vi "pf_Config_and_Grab.vi"() -> ()   [LabVIEW 2012]
uses:
  <userlib>/Photonfocus Toolkit/_Public/SubVIs/pf_Set_Camera_Property_Float.vi
  <userlib>/Photonfocus Toolkit/_Public/SubVIs/pf_Set_Camera_Property_Mode.vi
  <userlib>/Photonfocus Toolkit/_Public/SubVIs/pf_Set_Camera_Property_Int.vi
  <userlib>/Photonfocus Toolkit/Photonfocus_Toolkit.lvlib
panel:
  in  "stop":bool
  in  "Tab Control":enum32{"Instructions", "image"}(tab)
  in  "Interface Name":string="img0::0||port0"
  out "Image":T1(plugin-control)
  # "1 - Open MAX and specify the correct .icd file."
  # "2 - Get the interface name from MAX (e.g: \"imag0\") and write it in the following text field. \n\n3 - Add \"::\" and the Port number showed in MAX.\n\n4 - Add \"||\" and the port name showed in PFRemote."
  # "::"
  # "||port0"
  # "Example:   img0::0||port0"
  # "5 - Close MAX before start grabbing"
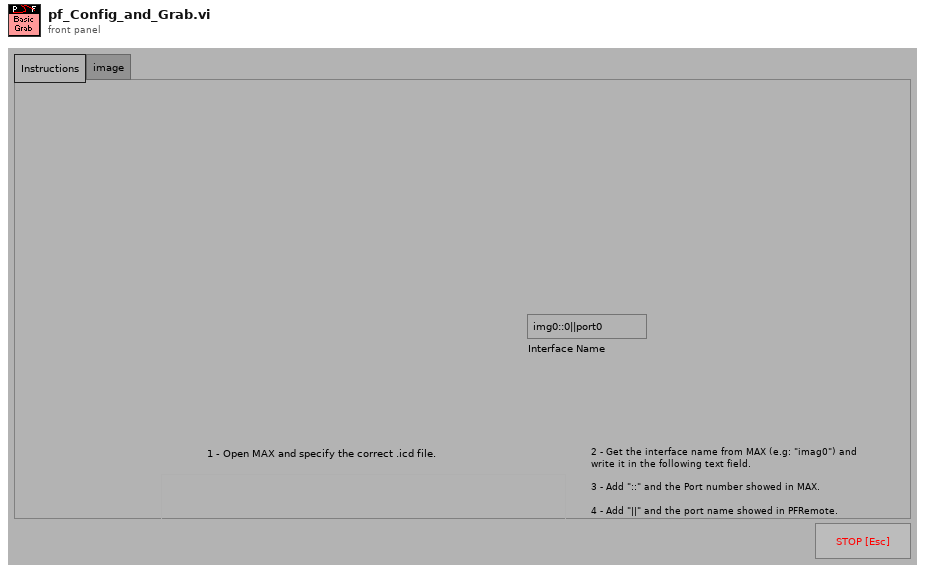
[diagram p1: front panel]
types:
  T1 = typedef "IMAQ Image.ctl" = refnum<image>
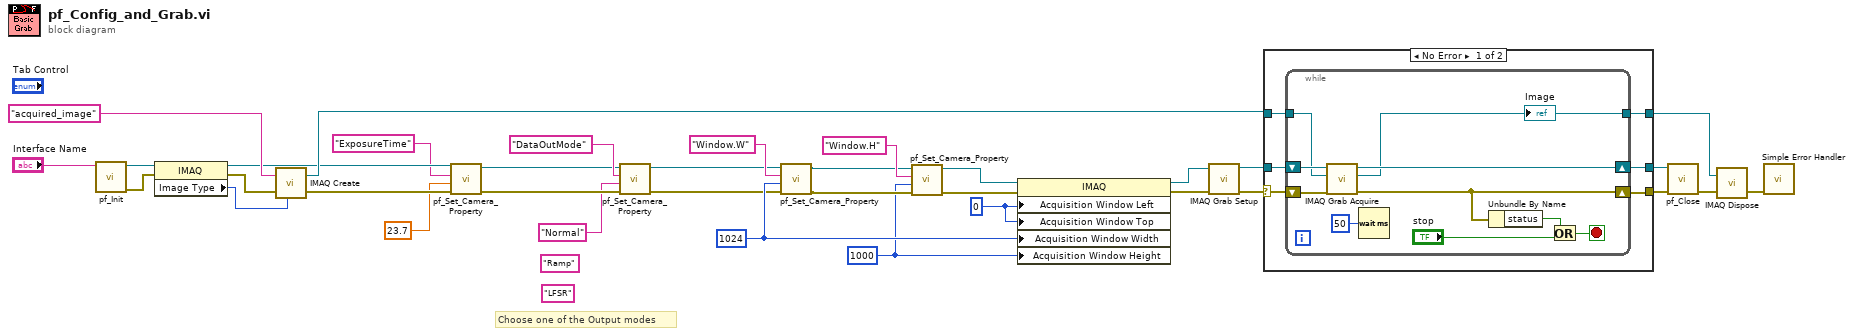
[diagram p0: block diagram]
diagram:
  w1 = u32 1000 ("milliseconds to wait")
  w15 = u32 0 ("milliseconds to wait")
  (unwired) "Ramp" ("Property Value")
  (unwired) "LFSR" ("Property Value")
  w7 = u32 1024 ("milliseconds to wait")
  # "Choose one of the Output modes"
  n1 = call <userlib>:"pf_Init.vi"("Interface Name"="Interface Name") -> ("error out"=w28:errorcluster, "IMAQ Session out"=w29:refnum<k11>)  [unwired: 2 in, 7 out]
  n2 = property class="IMAQ"(reference=w29, error in=w28) -> (reference out=w20:refnum<k11>, error out=w34:errorcluster, "Image Type"=w35:u32)
  n3 = call "IMAQ Create"("Image Name"="acquired_image", "Image Type"=w35, "error in (no error)"=w34) -> ("New Image"=w22:T1, "error out"=w21:errorcluster)  [unwired: 1 in, 1 out]
  n4 = call-poly <userlib>:"pf_Set_Camera_Property.vi"("error in (no error)"=w21, "Property Value"=23.7 ("milliseconds to wait"), "Property Name"="ExposureTime" ("Image Name"), "IMAQ Session in"=w20) -> ("error out"=w6:errorcluster, "IMAQ Session out"=w4:refnum<k11>)  [unwired: 5 in, 1 out]
  n5 = call-poly <userlib>:"pf_Set_Camera_Property.vi"("error in (no error)"=w6, "Property Value"="Normal", "Property Name"="DataOutMode" ("Image Name"), "IMAQ Session in"=w4) -> ("error out"=w5:errorcluster, "IMAQ Session out"=w3:refnum<k11>)  [unwired: 5 in, 1 out]
  n6 = call-poly <userlib>:"pf_Set_Camera_Property.vi"("error in (no error)"=w5, "Property Value"=w7, "Property Name"="Window.W" ("Image Name"), "IMAQ Session in"=w3) -> ("error out"=w11:errorcluster, "IMAQ Session out"=w10:refnum<k11>)  [unwired: 5 in, 1 out]
  n7 = call-poly <userlib>:"pf_Set_Camera_Property.vi"("error in (no error)"=w11, "Property Value"=w1, "Property Name"="Window.H" ("Image Name"), "IMAQ Session in"=w10) -> ("error out"=w9:errorcluster, "IMAQ Session out"=w8:refnum<k11>)  [unwired: 5 in, 1 out]
  n8 = property class="IMAQ"(reference=w8, error in=w9, "Acquisition Window Left"=w15, "Acquisition Window Top"=w15, "Acquisition Window Width"=w7, "Acquisition Window Height"=w1) -> (reference out=w13:refnum<k11>, error out=w14:errorcluster)
  n9 = call <vilib>:"IMAQ Grab Setup.vi"("error in (no error)"=w14, "IMAQ Session In"=w13) -> ("error out"=w23:errorcluster, "IMAQ Session Out"=w25:refnum<k11>)  [unwired: 8 out]
  n10 = case shown="No Error" w23 {
    selector: w23 -> [w38 w54]
    tunnel: [w36 w54] -> w27
    tunnel: w22 -> [w41 w53]
    tunnel: [w40 w53] -> w31
    tunnel: w25 -> [w39 w52]
    tunnel: [w37 w52] -> w24
    frame No Error {
      n11 = while {
        tunnel: w41 -> [w43]
        tunnel: [w44] -> w40
        shift-right: [w42] -> w36
        shift-left: w38 -> [w46]
        shift-right: [w45] -> w37
        shift-left: w39 -> [w47]
        stop <- w48 stop-if-true
        n12 = call <vilib>:"IMAQ Grab Acquire.vi"("error in (no error)"=w46, "Image In"=w43, "IMAQ Session In"=w47) -> ("error out"=w42:errorcluster, "Image Out"=w44:T1, "IMAQ Session Out"=w45:refnum<k11>)  [unwired: 1 in, 5 out]
        "Image" <- w44
        n13 = Wait (ms)(milliseconds to wait=u32 50) -> ()  [unwired: 1 out]
        n14 = Unbundle By Name(w42) -> ("status"=w49:bool)
        n15 = Or(x=w49, y="stop") -> (x .or. y?=w48:bool)
      }
    }
    frame Error {
    }
  }
  n16 = call <userlib>:"pf_Close.vi"("error in (no error)"=w27, "IMAQ Session in"=w24) -> ("error out"=w26:errorcluster)  [unwired: 9 out]
  n17 = call "IMAQ Dispose"("Image"=w31, "error in (no error)"=w26) -> ("error out"=w33:errorcluster)  [unwired: 1 in, 3 out]
  n18 = call <vilib>:"Simple Error Handler.vi"("error in (no error)"=w33) -> ()  [unwired: 1 in, 8 out]
